vi "TCP Wait on listener.vi"(8 "error in (no error)":errorcluster, 9 "timeout ms (wait forever: -1)":i32=-1, 10 "resolve remote address (T)":bool=TRUE, 11 "TCP in":refnum<class "TCP.lvclass">) -> (0 "error out":errorcluster, 1 "remote port":u16, 2 "remote address":string, 3 "TCP out":refnum<class "TCP.lvclass">, 4 "connection ID":refnum<class "TCP.lvclass">)   [LabVIEW 2013, in "TCP.lvclass"]
doc: "Waits for an accepted TCP network connection"
uses:
  TCP.lvclass
  TCP.lvclass/TCP.ctl
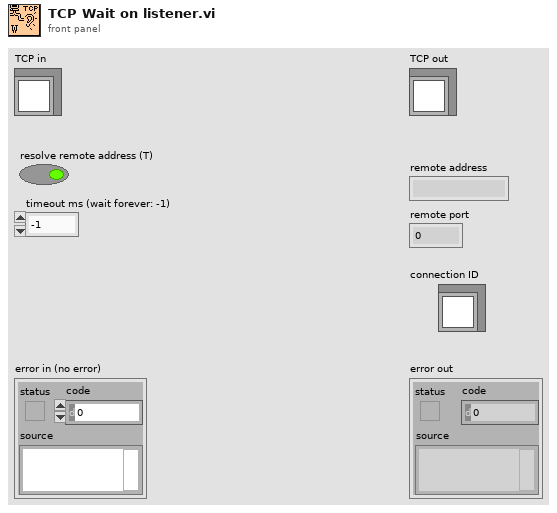
[diagram p1: front panel]
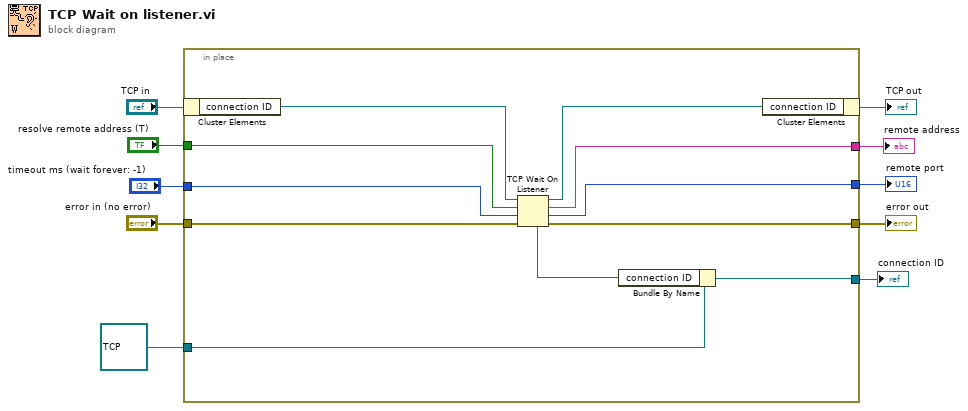
[diagram p0: block diagram]
diagram:
  n1 = in-place {
    in-place-border: "error in (no error)" -> [w19]
    in-place-border: [w18] -> w9
    in-place-border: [w16] -> w6
    in-place-border: refnum<class "TCP.lvclass"> refnum ("TCP in") -> [w15]
    in-place-border: [w14] -> w4
    in-place-border: [w13] -> w3
    in-place-border: "resolve remote address (T)" -> [w12]
    in-place-border: "timeout ms (wait forever: -1)" -> [w11]
    n2 = in-place-cluster #1("TCP in") -> ("connection ID"=w21:refnum<k5>)
    n3 = TCP Wait On Listener(8:w19, 9:w11, 10:w12, 11:w21) -> (0:w18:errorcluster, 1:w13:u16, 2:w14:string, 3:w20:refnum<k5>, 4:w17:refnum<k5>)
    n4 = Bundle By Name(cluster=w15, "connection ID"=w17) -> (w16:refnum<class "TCP.lvclass">)
    n5 = in-place-cluster #1("connection ID"=w20) -> (→"TCP out":refnum<class "TCP.lvclass">)
  }
  "error out" <- w9
  "connection ID" <- w6
  "remote address" <- w4
  "remote port" <- w3
